vi "test_notLaunchedTaskShouldReturnNoError.vi"(11 "Test Case In":refnum<class "TaskControllerTests.lvclass">) -> (0 "error out":errorcluster, 3 "Test Case Out":refnum<class "TaskControllerTests.lvclass">)   [LabVIEW 2023, in "TaskControllerTests.lvclass"]
uses:
  <vilib>/Astemes/LUnit/Test Case.lvclass/Test Case.ctl
  <vilib>/Astemes/LUnit/Core/LUnit Test Case/Private/Append Fail Result.vi
  <vilib>/Astemes/LUnit/Core/LUnit Test Case/Private/Append Pass Result.vi
  <vilib>/Astemes/LUnit/Core/LUnit Test Case/Private/Run In UI.vi
  <vilib>/Utility/error.llb/Clear Errors.vi
  TaskMock/TaskMock.lvclass
  TaskControllerTests.lvclass
  TaskControllerTests.lvclass/TaskControllerTests.ctl
  source/TaskController/TaskController.lvclass
  <vilib>/Astemes/LUnit/Test Case.lvclass
  C:/projects/TLC_Daemon/tests/TaskMock/TaskMock.lvclass
  C:/projects/TLC_Daemon/source/ITask/ITask.lvclass
  C:/Program Files (x86)/National Instruments/LabVIEW 2023/vi.lib/Astemes/LUnit/Test Case.lvclass
  C:/Program Files (x86)/National Instruments/LabVIEW 2023/vi.lib/Astemes/LUnit/LUnit Runnable.lvclass
  C:/projects/TLC_Daemon/tests/TaskControllerTests/TaskControllerTests.lvclass
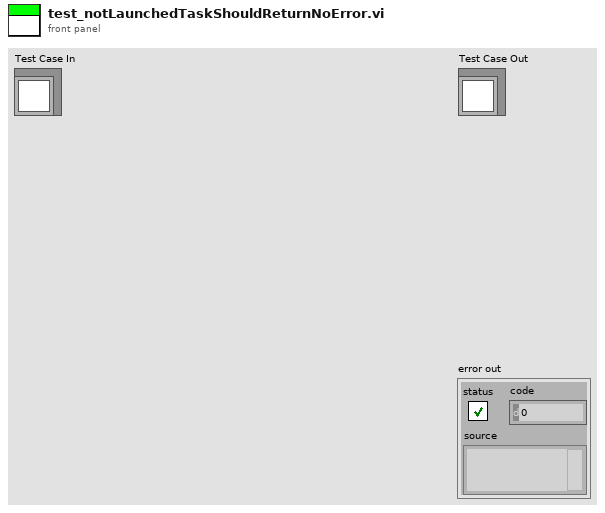
[diagram p1: front panel]
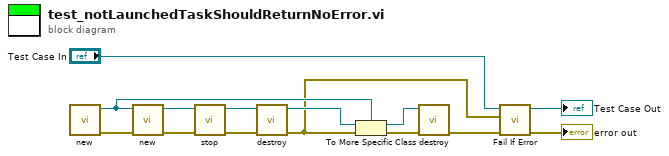
[diagram p0: block diagram]
diagram:
  n1 = call "new.vi"() -> ("error out"=w4:errorcluster, "TaskMock out"=w7:refnum<class "TaskMock.lvclass">)  [unwired: 10 in]
  n2 = call "new.vi"("error in (no error)"=w4, "task"=w7) -> ("error out"=w10:errorcluster, "TaskController out"=w11:refnum<class "TaskController.lvclass">)  [unwired: 8 in]
  n3 = call "stop.vi"("error in (no error)"=w10, "TaskController in"=w11) -> ("error out"=w8:errorcluster, "TaskController out"=w9:refnum<class "TaskController.lvclass">)  [unwired: 8 in]
  n4 = call "destroy.vi"("error in (no error)"=w8, "TaskController in"=w9) -> ("error out"=w1:errorcluster, "taskResult"=w6:refnum<class "ITask.lvclass">)  [unwired: 8 in]
  n5 = To More Specific Class(target class=w7, reference=w6, error in=w1) -> (specific class reference=w5:refnum<class "TaskMock.lvclass">, error out=w2:errorcluster)
  n6 = call "destroy.vi"("error in (no error)"=w2, "TaskMock in"=w5) -> ("error out"=w3:errorcluster)  [unwired: 9 in]
  n7 = call <vilib>:"Fail If Error.vi"("error in (no error)"=w3, "Assert error"=w1, "LUnit Test Case In"="Test Case In") -> ("error out"=→"error out":errorcluster, "LUnit Test Case Out"=→"Test Case Out":refnum<class "TaskControllerTests.lvclass">)  [unwired: 7 in]
